vi "connect.vi"(0 "PI_Piezo.lvclass (in)":refnum<class "PI_Piezo.lvclass">, 11 "error in":errorcluster) -> (4 "PI_Piezo.lvclass":refnum<class "PI_Piezo.lvclass">, 15 "error out":errorcluster)   [LabVIEW 2013, in "PI_Piezo.lvclass"]
doc: "This VI demonstrates how to initialize an E-816 system with more than one axis, how to move all connected axes and how to query for the position value. \n\nIn this example the E-816 is connected through USB. The Serial No. of the system to command is not known, so the \"Search for controllers\" control is left TRUE. The VI runs E816_Configuration_Setup.vi with specified settings, moves the connected axes relative to their current position, waits for the movement to finish and reads the position of the axes and the error status of the controller. Instead of calling the corresponding command VIs, it uses \"Split multiple axes command.vi\" which sends the chosen commands for the given axes one after another and returns the answer array (if any). The diagram shows how to combine the driver VIs for these tasks. \n\nFor an example of how to command a single axis E-816 system connected through RS-232 see E816_Sample_ Application_1.vi\n\nWarning: Before running this VI, modify the interface settings on the block diagram to reflect your configuration. The predefined settings provided with the VI probably do not match your system."
uses:
  PI_Piezo.lvclass
  PI_Piezo.lvclass/PI_Piezo.ctl
  Globals.vi
panel:
  # "This VI demonstrates how to initialize an E-816 system with more than one axis, how to move all connected axes and how to query\nfor the position value. The VI runs E816_Configuration_Setup.vi with specified settings, moves the connected axes relative to their \ncurrent position and reads the position. Instead of calling the corresponding command VIs, it uses \"Split multiple axes command.vi\"\nwhich sends the chosen commands for the given axes one after another and returns the answer array (if any). The diagram shows\nhow to combine the driver VIs for these tasks. \n\nWarning: Before running this VI, modify the interface settings on the block diagram to reflect your configuration. The predefined \n                 settings provided with the VI probably do not match your system."
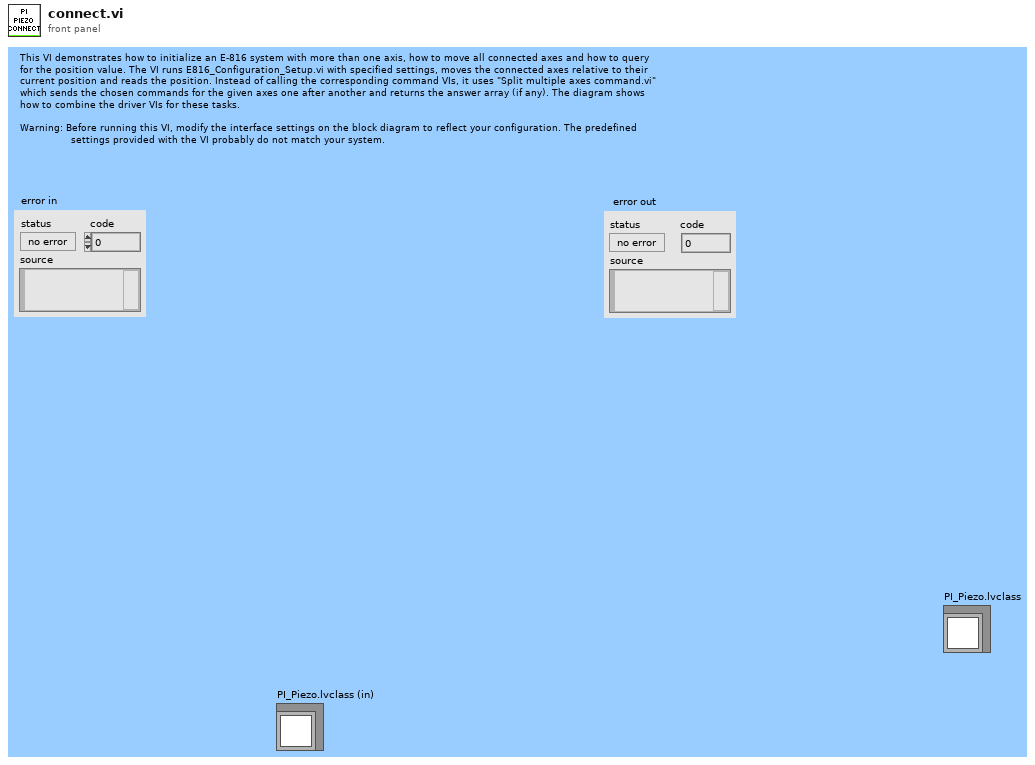
[diagram p1: front panel]
types:
  T1 = enum16{"DCO", "DCO?", "MOV", "MOV?", "MVR", "ONT?", "OVF?", "POS?", "RST", "SVA", "SVA?", "SVO", "SVO?", "SVR", "VOL?", "GWait"}
  T2 = typedef "PI_Piezo.lvclass/settings.ctl" = cluster{"Enable":bool, "Array of Piezo Controllers":T3[]}
  T3 = typedef "PI_Piezo.lvclass/piezo_controller.ctl" = cluster{"Enable":bool, "Serial No.":string, "Array of Piezo Channels":T4[]}
  T4 = typedef "PI_Piezo.lvclass/piezo_channel.ctl" = cluster{"Servo":bool, "Set Position":dbl}
  T5 = cluster{"Axis":string, "Servo":bool, "Position":dbl}
  T6 = cluster{"Identification":string, "SN out":string, cluster{"Axis":string, "Servo":bool, "Position":dbl}[]}
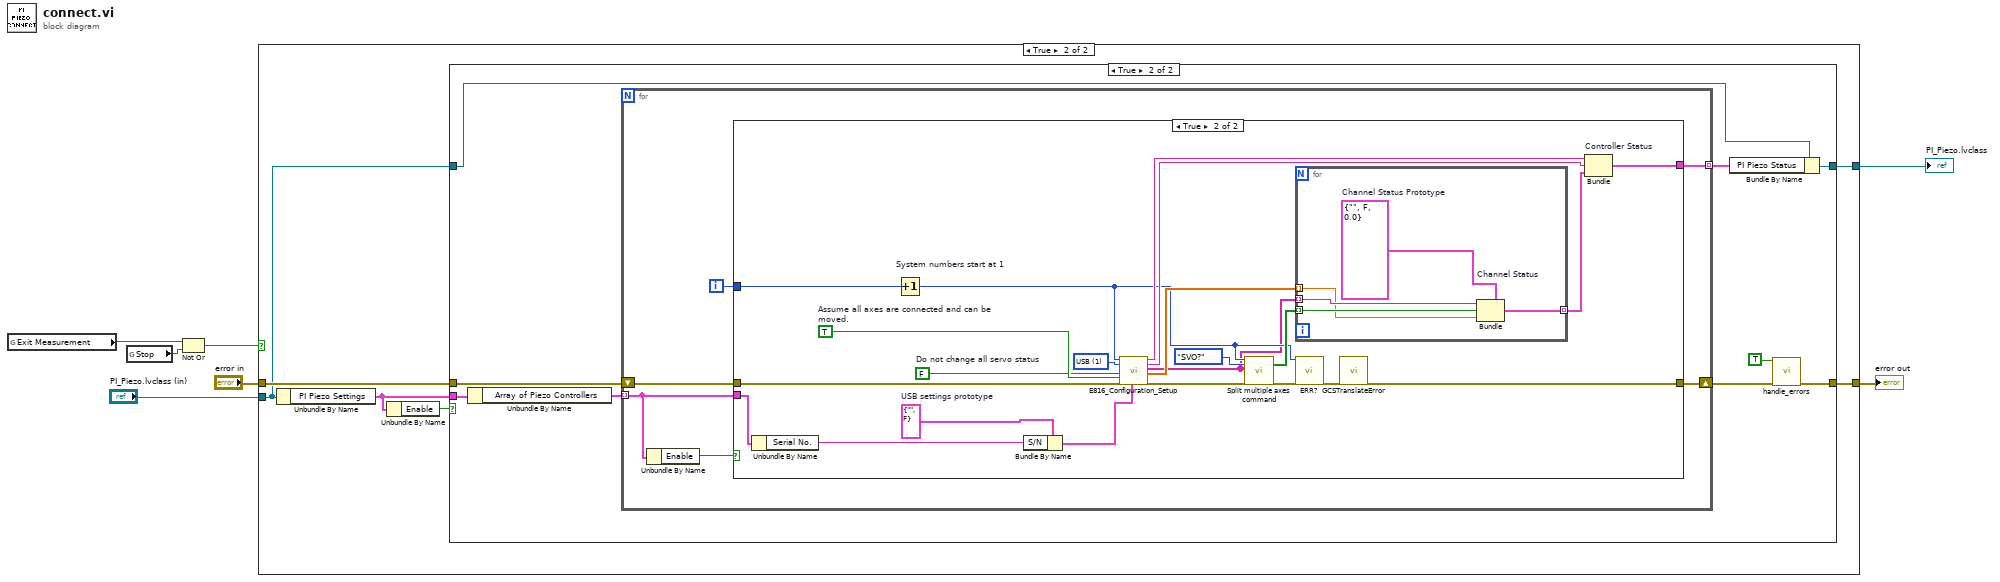
[diagram p0: block diagram]
diagram:
  n1 = global read "Globals.vi" "Exit Measurement"() -> (w3:bool)
  n2 = global read "Globals.vi" "Stop"() -> (w2:bool)
  n3 = Not Or(1:w2, 2:w3) -> (0:w1:bool)
  n4 = case shown="True" w1 {
    tunnel: "error in" -> [w9 w14]
    tunnel: [w8 w12] -> w6
    tunnel: "PI_Piezo.lvclass (in)" -> [w8 w11]
    tunnel: [w9 w10] -> w4
    frame False {
    }
    frame True {
      n5 = Unbundle By Name(w11) -> ("PI Piezo Settings"=w13:T2)
      n6 = Unbundle By Name(w13) -> ("Enable"=w15:bool)
      n7 = case shown="True" w15 {
        tunnel: w13 -> [_ w26]
        tunnel: w14 -> [w17 w24]
        tunnel: [w17 w18] -> w10
        tunnel: [w16 w23] -> w12
        tunnel: w11 -> [w16 w22]
        frame False {
        }
        frame True {
          n8 = Unbundle By Name(w26) -> ("Array of Piezo Controllers"=w25:T3[])
          n9 = for {
            tunnel: w25 -> [w30] mode=indexing
            shift-right: [w28] -> w19
            shift-left: w24 -> [w29]
            tunnel: [w27] -> w21 mode=indexing
            i -> [w31]
            n10 = Unbundle By Name(w30) -> ("Enable"=w32:bool)
            n11 = case shown="True" w32 {
              tunnel: w31 -> [_ w55]
              tunnel: w30 -> [_ w53]
              tunnel: w29 -> [w33 w48]
              tunnel: [w33 w42] -> w28
              tunnel: [_ w45] -> w27
              frame False {
              }
              frame True {
                w44 = TRUE  # Assume all axes are connected and can be moved.
                w49 = FALSE  # Do not change all servo status
                w51 = cluster{"S/N":string, "USB Search?":bool} {"S/N"="", "USB Search?"=FALSE}  # USB settings prototype
                w54 = u16 1 items=["RS232", "USB"] ("Interface")
                n12 = Unbundle By Name(w53) -> ("Serial No."=w52:string)
                n13 = Increment "System numbers start at 1"(x=w55) -> (x+1=w37:i32)
                n14 = Bundle By Name(cluster=w51, "S/N"=w52) -> (w50:cluster{"S/N":string, "USB Search?":bool})
                n15 = call "E816_Configuration_Setup.vi"("System no."=w37, "Interface"=w54, "All axes?"=w44, "Change servo \nstatus to ON?"=w49, "error in"=w48, "USB settings"=w50) -> ("Identification"=w47:string, "SN out"=w46:string, "Conn. Axes"=w36:string[], "Position"=w40:dbl[], "error out"=w35:errorcluster)  [unwired: 9 in]
                n16 = call "Split multiple axes command.vi"("System no."=w37, "Command"=T1."SVO?", "Axes to command"=w36, "error in"=w35) -> ("Bool. values out"=w38:bool[], "error out"=w34:errorcluster)  [unwired: 13 in, 1 out]
                n17 = for {
                  tunnel: w38 -> [w60] mode=indexing
                  tunnel: [w59] -> w41 mode=indexing
                  tunnel: w36 -> [w58] mode=indexing
                  tunnel: w40 -> [w56] mode=indexing
                  w57 = T5 {"Axis"="", "Servo"=FALSE, "Position"=0.0}  # Channel Status Prototype
                  n18 = Bundle "Channel Status"(cluster=w57, "Axis"=w58, "Servo"=w60, "Position"=w56) -> (w59:T5)
                }
                n19 = call "ERR?.vi"("System no."=w37, "error in"=w34) -> ("error out"=w43:errorcluster)  [unwired: 16 in, 1 out]
                n20 = call "GCSTranslateError.vi"("error in"=w43) -> ("error out"=w42:errorcluster)  [unwired: 16 in, 2 out]
                n21 = Bundle "Controller Status"("Identification"=w47, "SN out"=w46, w41) -> (w45:T6)  [unwired: 1 in]
              }
            }
          }
          n22 = Bundle By Name(cluster=w22, "PI Piezo Status"=w21) -> (w23:refnum<class "PI_Piezo.lvclass">)
          n23 = call "handle_errors.vi"("Exit Operation"=TRUE ("Exit Measurement"), "error in (no error)"=w19) -> ("error out"=w18:errorcluster)  [unwired: 13 in]
        }
      }
    }
  }
  "PI_Piezo.lvclass" <- w6
  "error out" <- w4
